vi "cmc-inclass-identitymatrix.vi"() -> ()   [LabVIEW 2010]
uses:
  <vilib>/Analysis/Matrix/Datatypes/RealMatrix.ctl
  <vilib>/Analysis/Matrix/NI_Matrix.lvlib
panel:
  in  "Matrix Size":dbl
  out "Real Matrix":T1
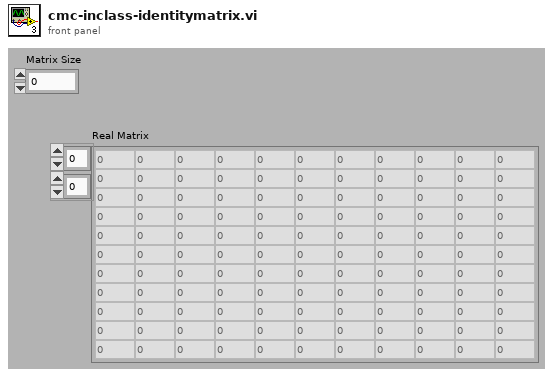
[diagram p1: front panel]
types:
  T1 = typedef "NI_Matrix.lvlib/RealMatrix.ctl" = dbl[][]
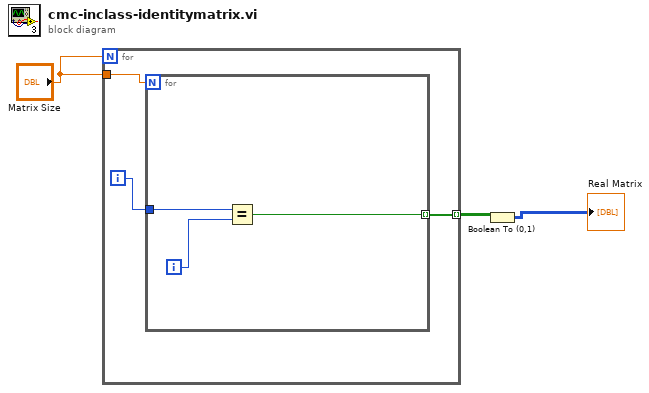
[diagram p0: block diagram]
diagram:
  n1 = for {
    N: "Matrix Size" -> [_]
    tunnel: "Matrix Size" -> [w6]
    tunnel: [w4] -> w2 mode=indexing
    i -> [w5]
    n2 = for {
      N: w6 -> [_]
      tunnel: w5 -> [w9]
      tunnel: [w7] -> w4 mode=indexing
      i -> [w8]
      n3 = Equal?(x=w9, y=w8) -> (x = y?=w7:bool)
    }
  }
  n4 = Boolean To (0,1)(Boolean=w2) -> (0, 1=→"Real Matrix":i16[][])
